vi "WS1021 RFFE Multi Dut Handshake Check.vi"(0 "HS CHK CNTRL":string[](array[string])=["01", "02", "04", "08", "03", "06", "0C", "07", "0E", "0F", "07", "03", "00"], 1 "TMN DC\\CAP Data Log File Path":path, 2 "Debug?":bool, 5 "Set Register":string="3", 6 "Select Brd":enum16{"A", "B"}(ring), 7 "Lot#":string="1K3CB", 8 "Stop Button":bool, 9 "Wafer #":string="9", 10 "File Name":string, 11 "Error In":errorcluster, 12 "FPGA":T2, 13 "SN#":string[](array[string]), 14 "Start":bool) -> (3 "Status":string[](array[string]), 4 "Pass/Fail?":bool[](array[boolean]), 15 "Error Out":errorcluster)   [LabVIEW 2017]
uses:
  WS_VCAP Driver 039/Source/WSVCAP Shell/Type Defs/WSVCAP SHL FPGA Enum.ctl
  <vilib>/userdefined/High Color/nirio_resource_hc.ctl
panel:
  in  "RFFE Slave Address":u8=7 caption="Slave Address" format="0x%02x"
  in  "Clock Rate Meas(Hz)":dbl=1000000.0 format="%.1p Hz"
  in  "Comment":string="HS-CHK"
  out "Simulate FPGA":bool
  out "Online":bool
  out "FPGA Resource":T1
  out "Activity Log":string
  out "P/F":string
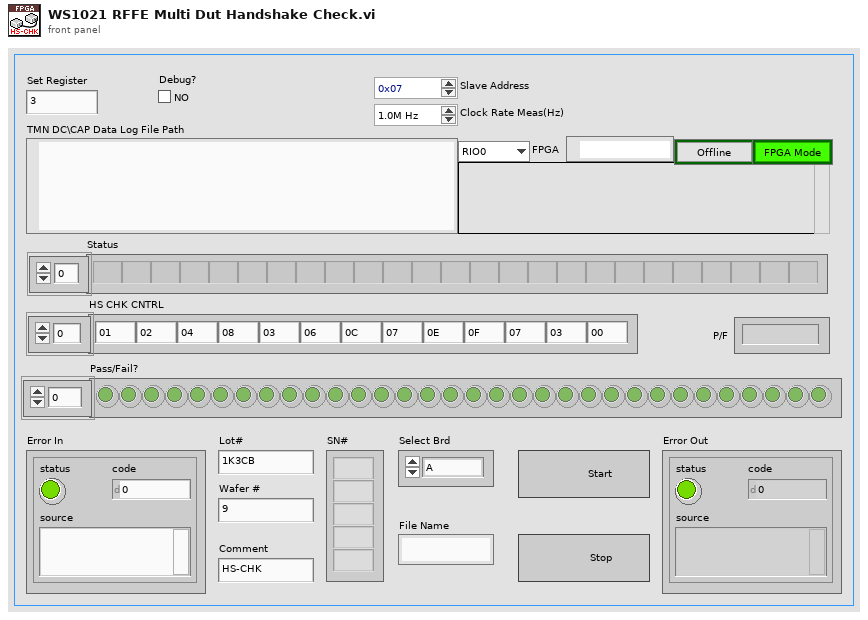
[diagram p1: front panel]
types:
  T1 = typedef "nirio_resource_hc.ctl" = tag
  T2 = typedef "WSVCAP SHL FPGA Enum.ctl" = enum16{"RIO0", "RIO1"}
  T3 = typedef "WSVCAP SHL Core System Cluster.ctl" = cluster{"Settings":T4, "FPGA Resource":tag, "Online":bool, "I2C Wait Ticks":u32, "SPI Wait Ticks":u32, "RFFE Wait Ticks":u32, "FPGA VI Reference (FPGA Mode)":T5, "FPGA VI Reference (Sim Mode)":refnum<vi>}
  T4 = typedef "WSVCAP SHL I2C Settings Cluster.ctl" = cluster{"I2C Slave Address":u8, "I2C Clock Rate (Hz)":dbl, "SPI Clock Rate (Hz)":dbl, "RFFE Slave Address":u8, "RFFE Clock Rate (Hz)":dbl, "Simulate FPGA":bool, "C1 Cap DAC Default":u8, "C2 Cap DAC Default":u8, "C3 Cap DAC Default":u8, "C4 Cap DAC Default":u8}
  T5 = typedef "WSVCAP SHL FPGA Ref.ctl" = refnum<k20>
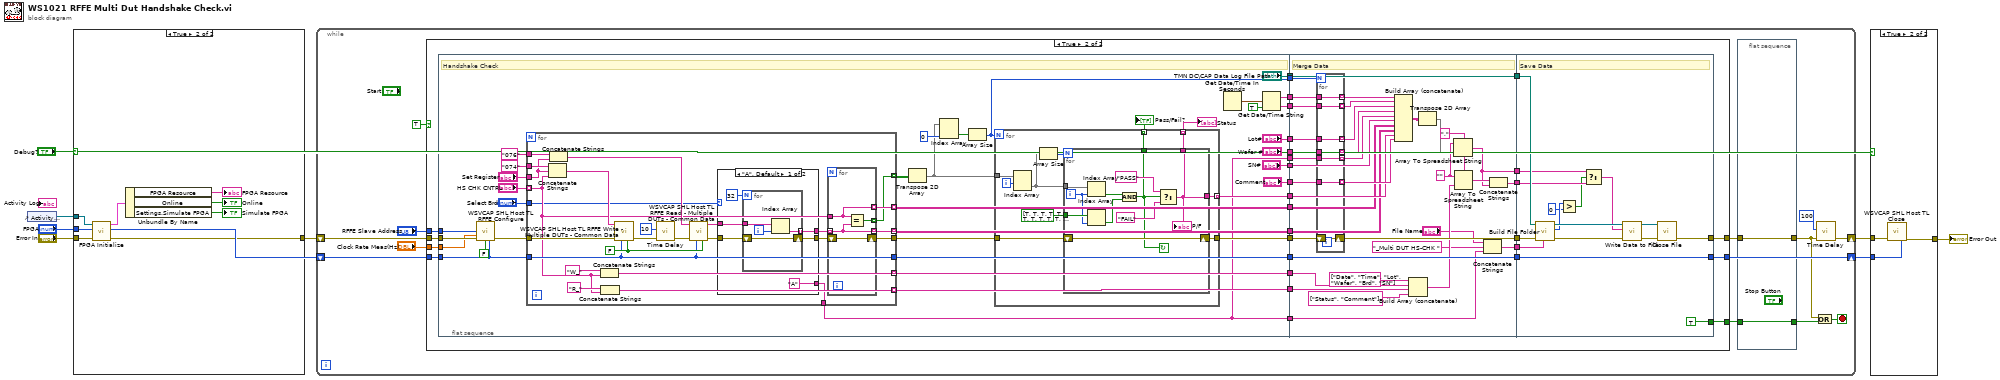
[diagram p0: block diagram]
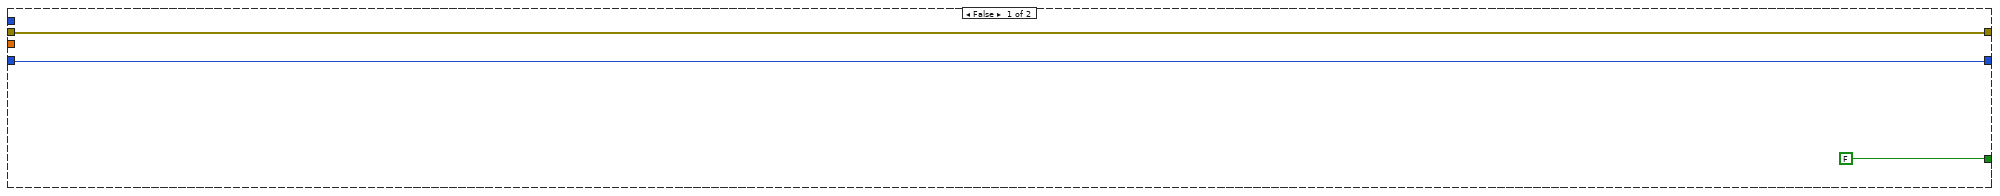
[diagram p2: hidden frame]
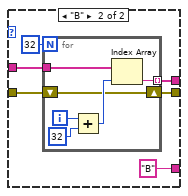
[diagram p3: hidden frame]
diagram:
  n1 = control-ref of="Activity Log"() -> (w7:refnum<vi>)
  n2 = case shown="True" "Debug?" {
    tunnel: "Error In" -> [w9 w17]
    tunnel: "FPGA" -> [_ w16]
    tunnel: w7 -> [_ w15]
    tunnel: [w9 w10] -> w6
    frame False {
    }
    frame True {
      n3 = call "FPGA Initialize.vi"("Error In"=w17, "FPGA"=w16, "Active Log"=w15) -> ("Error Out"=w10:errorcluster, "System Out"=w14:T3)  [unwired: 7 in]
      n4 = Unbundle By Name(w14) -> ("FPGA Resource"=→"FPGA Resource":tag, "Online"=→"Online":bool, "Settings.Simulate FPGA"=→"Simulate FPGA":bool)
    }
  }
  n5 = while {
    shift-right: [w26] -> w3
    shift-left: w6 -> [w30]
    shift-right: [w28] -> w4
    shift-left: "FPGA" -> [w29]
    stop <- w27 stop-if-true
    n6 = case shown="True" TRUE {
      tunnel: w30 -> [w34 w65]
      tunnel: w29 -> [w35 w64]
      tunnel: [w35 w63] -> w28
      tunnel: [w34 w62] -> w24
      tunnel: [FALSE w41] -> w21
      tunnel: "RFFE Slave Address" -> [_ w40]
      tunnel: "Clock Rate Meas(Hz)" -> [_ w39]
      frame False {
      }
      frame True {
        n7 = flat-sequence {
          tunnel: w65 -> [w73]
          tunnel: w64 -> [w69]
          tunnel: [w95] -> w61
          tunnel: [w86] -> w60
          tunnel: [w91] -> w59
          tunnel: [w90] -> w58
          tunnel: ["Lot#"] -> w57
          tunnel: ["Wafer #"] -> w56
          tunnel: ["SN#"] -> w55
          tunnel: [w85] -> w54
          tunnel: [w84] -> w53
          tunnel: ["TMN DC\\CAP Data Log File Path"] -> w49
          tunnel: [w82] -> w45
          tunnel: ["Comment"] -> w44
          tunnel: [w80] -> w43
          tunnel: [w79] -> w42
          tunnel: w40 -> [w71]
          tunnel: w39 -> [w70]
          tunnel: [w68] -> w38
          tunnel: [w66] -> w37
          tunnel: [w66] -> w36
          tunnel: w61 -> [w210]
          tunnel: w60 -> [w209]
          tunnel: w59 -> [w208]
          tunnel: w58 -> [w207]
          tunnel: w57 -> [w200]
          tunnel: w56 -> [w199]
          tunnel: w55 -> [w176]
          tunnel: w54 -> [w177]
          tunnel: w53 -> [w178]
          tunnel: [w210] -> w52
          tunnel: [w202] -> w51
          tunnel: [w201] -> w50
          tunnel: w49 -> [w201]
          tunnel: [w184] -> w48
          tunnel: [w193] -> w47
          tunnel: [w192] -> w46
          tunnel: w45 -> [w179]
          tunnel: w44 -> [w191]
          tunnel: w43 -> [w189]
          tunnel: w42 -> [w188]
          tunnel: w38 -> [w185]
          tunnel: w37 -> [w182]
          tunnel: w36 -> [w181]
          tunnel: [w229] -> w62
          tunnel: [w233] -> w63
          tunnel: w52 -> [w233]
          tunnel: w51 -> [w232]
          tunnel: w50 -> [w231]
          tunnel: w48 -> [w230]
          tunnel: w47 -> [w221]
          tunnel: w46 -> [w222]
          tunnel: [TRUE] -> w41
          frame #0 {
            # "Handshake Check"
            n8 = call "WSVCAP SHL Host TL RFFE Configure.vi"("RFFE Slave Address"=w71, "Clock Rate (Hz)"=w70, "error in"=w73, "Log (T)"=FALSE, "FPGA"=w69) -> ("error out"=w72:errorcluster)  [unwired: 9 in, 1 out]
            n9 = for {
              tunnel: "HS CHK CNTRL" -> [w131] mode=indexing
              tunnel: "Set Register" -> [w133]
              tunnel: "074" ("string") -> [w147]
              tunnel: w69 -> [w137]
              tunnel: "076" ("string") -> [w142]
              tunnel: w72 -> [w140]
              tunnel: [w128] -> w78 mode=indexing
              tunnel: [w138] -> w97
              tunnel: [w137] -> w95
              tunnel: [w136] -> w85 mode=indexing
              tunnel: [w135] -> w84 mode=indexing
              tunnel: [w130] -> w80 mode=indexing
              tunnel: [w129] -> w79 mode=indexing
              tunnel: "Select Brd" -> [w127]
              tunnel: [w122] -> w66
              w139 = FALSE ("Log (T)")
              n10 = Concatenate Strings(w147, w133, w131) -> (w146:string)
              n11 = Concatenate Strings(w142, w133) -> (w141:string)
              n12 = Concatenate Strings("W_" ("string"), w131) -> (w130:string)
              n13 = Concatenate Strings("R_" ("string"), w131) -> (w129:string)
              n14 = call "WSVCAP SHL Host TL RFFE Write - Multiple DUTs - Common Data.vi"("Data Out"=w146, "error in"=w140, "FPGA"=w137, "Log (T)"=w139) -> ("error out"=w145:errorcluster)  [unwired: 11 in]
              n15 = call "Time Delay.vi"("Error In"=w145, "Delay(ms)"=u32 10) -> ("Error Out"=w144:errorcluster)  [unwired: 9 in]
              n16 = call "WSVCAP SHL Host TL RFFE Read - Multiple DUTs - Common Data.vi"("Data Out"=w141, "error in"=w144, "FPGA"=w137, "Log (T)"=w139) -> ("RFFE Data In"=w125:string[], "error out"=w126:errorcluster)  [unwired: 10 in]
              n17 = case shown="\"A\", Default" w127 {
                tunnel: w126 -> [w150 w161]
                tunnel: w125 -> [w152 w162]
                tunnel: [w151 w160] -> w124
                tunnel: [w149 w159] -> w123
                tunnel: ["A" "B"] -> w122
                frame "A", Default {
                  n18 = for {
                    N: 32 -> [_]
                    tunnel: w152 -> [w157]
                    tunnel: [w155] -> w151 mode=indexing
                    shift-right: [w154] -> w149
                    shift-left: w150 -> [w154]
                    i -> [w156]
                    n19 = Index Array(array=w157, index=w156) -> (element=w155:string)
                  }
                }
                frame "B" {
                  n20 = for {
                    N: 32 -> [_]
                    tunnel: w162 -> [w169]
                    tunnel: [w165] -> w160 mode=indexing
                    shift-right: [w164] -> w159
                    shift-left: w161 -> [w164]
                    i -> [w168]
                    n21 = Add(x=w168, y=32) -> (x+y=w166:i32)
                    n22 = Index Array(array=w169, index=w166) -> (element=w165:string)
                  }
                }
              }
              n23 = for {
                shift-right: [w173] -> w138
                shift-left: w123 -> [w173]
                tunnel: w124 -> [w170] mode=indexing
                tunnel: w131 -> [w171]
                tunnel: [w172] -> w128 mode=indexing
                tunnel: [w171] -> w136 mode=indexing
                tunnel: [w170] -> w135 mode=indexing
                n24 = Equal?(x=w171, y=w170) -> (x = y?=w172:bool)
              }
            }
            n25 = Transpose 2D Array(2D array=w78) -> (transposed array=w75:bool[][])
            n26 = Index Array(array=w75, index (col)=0 ("disabled index (col)")) -> (element=w76:bool[])  [unwired: 1 in]
            n27 = Array Size(array=w76) -> (size(s)=w68:i32)
            n28 = for {
              N: w68 -> [_]
              tunnel: w75 -> [w111]
              tunnel: w97 -> [w105]
              tunnel: [w106] -> w96 mode=indexing
              tunnel: [w104] -> w86
              tunnel: [w103] -> w94 mode=indexing
              tunnel: [w102] -> w82 mode=indexing
              i -> [w110]
              n29 = Index Array(array=w111, index (row)=w110) -> (element=w108:bool[])  [unwired: 1 in]
              n30 = Array Size(array=w108) -> (size(s)=w109:i32)
              n31 = for {
                N: w109 -> [_]
                tunnel: w108 -> [w121]
                tunnel: bool[] [TRUE, TRUE, TRUE, TRUE, TRUE, TRUE, TRUE, TRUE, TRUE, TRUE, TRUE, TRUE, TRUE, TRUE, TRUE, TRUE, TRUE, TRUE, TRUE, TRUE, TRUE, TRUE, TRUE, TRUE, TRUE, TRUE, TRUE, TRUE, TRUE, TRUE, TRUE, TRUE, TRUE, TRUE, TRUE, TRUE, TRUE, TRUE, TRUE, TRUE, TRUE, TRUE, TRUE, TRUE, TRUE, TRUE, TRUE, TRUE, TRUE, TRUE, TRUE, TRUE, TRUE, TRUE, TRUE, TRUE, TRUE, TRUE, TRUE, TRUE, TRUE, TRUE, TRUE, TRUE, TRUE, TRUE, TRUE, TRUE, TRUE, TRUE, TRUE, TRUE] -> [w120]
                tunnel: [w112] -> w106
                shift-right: [w114] -> w104
                shift-left: w105 -> [w114]
                tunnel: [w113] -> w103
                tunnel: [w112] -> w102
                i -> [w119]
                stop <- w113 continue-if-true
                n32 = Index Array(array=w121, index=w119) -> (element=w118:bool)
                n33 = Index Array(array=w120, index=w119) -> (element=w117:bool)
                n34 = And(x=w118, y=w117) -> (x .and. y?=w113:bool)
                n35 = Select(t="PASS", s=w113, f="FAIL") -> (s? t:f=w112:string)
                "P/F" <- w112
              }
            }
            "Pass/Fail?" <- w94
            "Status" <- w96
            n36 = Get Date/Time In Seconds() -> (seconds since 1Jan1904=w93:timestamp)
            n37 = Get Date/Time String(seconds (now)=w93, want seconds? (F)=TRUE) -> (date string=w91:string, time string=w90:string)  [unwired: 1 in]
          }
          frame #1 {
            w195 = "" ("format string")
            w196 = "," ("delimiter (Tab)")
            # "Merge Data"
            n38 = for {
              N: w185 -> [_]
              shift-right: [w217] -> w202
              shift-left: w209 -> [w217]
              tunnel: w208 -> [w213]
              tunnel: w207 -> [w214]
              tunnel: w200 -> [w216]
              tunnel: w199 -> [w215]
              tunnel: [w216] -> w204 mode=indexing
              tunnel: [w215] -> w203 mode=indexing
              tunnel: [w214] -> w205 mode=indexing
              tunnel: [w213] -> w206 mode=indexing
              tunnel: [w212] -> w180 mode=indexing
              tunnel: w191 -> [w212]
              tunnel: w181 -> [w211]
              tunnel: [w211] -> w175 mode=indexing
            }
            n39 = Build Array (concatenate)(w206, w205, w204, w203, w175, w176, w177, w178, w179, w180) -> (w198:string[][])
            n40 = Build Array (concatenate)(string[] ["Date", "Time", "Lot", "Wafer", "Brd", "SN"], w189, w188, string[] ["Status", "Comment"] ("array")) -> (w186:string[])
            n41 = Transpose 2D Array(2D array=w198) -> (transposed array=w194:string[][])
            n42 = Array To Spreadsheet String(delimiter (Tab)=w196, array=w194, 3:w195) -> (spreadsheet string=w192:string)
            n43 = Array To Spreadsheet String(delimiter (Tab)=w196, array=w186, 3:w195) -> (spreadsheet string=w197:string)
            n44 = Concatenate Strings("File Name", "_Multi DUT HS-CHK " ("Data format"), w182) -> (w184:string)
            n45 = Concatenate Strings(w197, w192) -> (w193:string)
          }
          frame #2 {
            # "Save Data"
            n46 = call "Build File Folder.vi"("File Name"=w230, "error in (no error)"=w232, "TMN DC\\CAP Data Log File Path"=w231) -> ("error out"=w225:errorcluster, "size (in bytes)"=w224:i64, "Byte Stream File out"=w226:refnum<file>)  [unwired: 6 in]
            n47 = Greater?(x=w224, y=i64 0) -> (0:w220:bool)
            n48 = Select(t=w222, s=w220, f=w221) -> (s? t:f=w219:string)
            n49 = call "Write Data to File.vi"("error in (no error)"=w225, "Data In"=w219, "File in"=w226) -> ("error out"=w227:errorcluster, "File out"=w228:refnum<file>)  [unwired: 7 in]
            n50 = call "Close File.vi"("error in"=w227, "File in"=w228) -> ("error out"=w229:errorcluster)  [unwired: 9 in]
          }
        }
      }
    }
    n51 = flat-sequence {
      tunnel: w24 -> [w32]
      tunnel: [w32] -> w23
      tunnel: [w31] -> w22
      tunnel: w21 -> [w31]
      frame #0 {
      }
    }
    n52 = Or(x=w23, y=w22) -> (x .or. y?=w27:bool)
    n53 = call "Time Delay.vi"("Error In"=w23, "Delay(ms)"=u32 100) -> ("Error Out"=w26:errorcluster)  [unwired: 9 in]
  }
  n54 = case shown="True" "Debug?" {
    tunnel: w4 -> [_ w237]
    tunnel: w3 -> [w234 w236]
    tunnel: [w234 w235] -> w2
    frame False {
    }
    frame True {
      n55 = call "WSVCAP SHL Host TL Close.vi"("error in"=w236, "FPGA"=w237) -> ("error out"=w235:errorcluster)  [unwired: 13 in]
    }
  }
  "Error Out" <- w2
